vi "voltCtrl.vi"() -> ()   [LabVIEW 2023]
uses:
  <vilib>/DAQmx/write.llb/DAQmx Write (Analog 1D DBL NChan 1Samp).vi
  <vilib>/DAQmx/create/channels.llb/DAQmx Create Channel (AO-Voltage-Basic).vi
  <vilib>/DAQmx/miscellaneous.llb/DAQmx Fill In Error Info.vi
panel:
  out "?":bool
  in  "crr":bool
  in  "Input":dbl(slide) scale=0.0..5.0
  in  "vltg":bool
  out "?":bool
  in  "?":bool
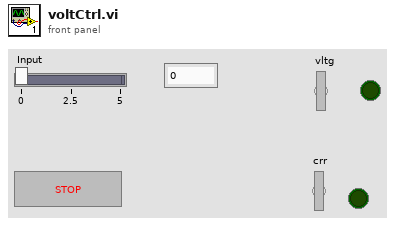
[diagram p1: front panel]
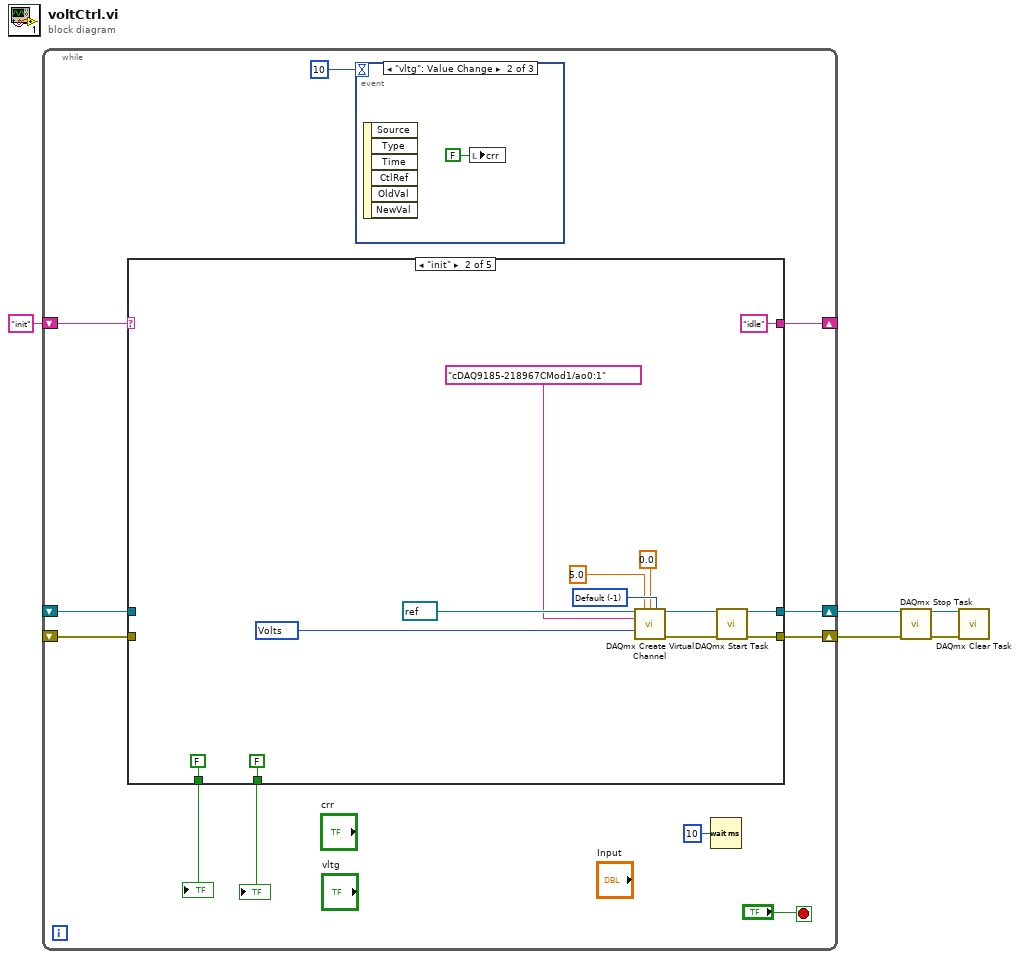
[diagram p0: block diagram]
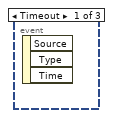
[diagram p2: hidden frame]
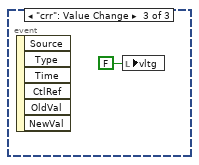
[diagram p3: hidden frame]
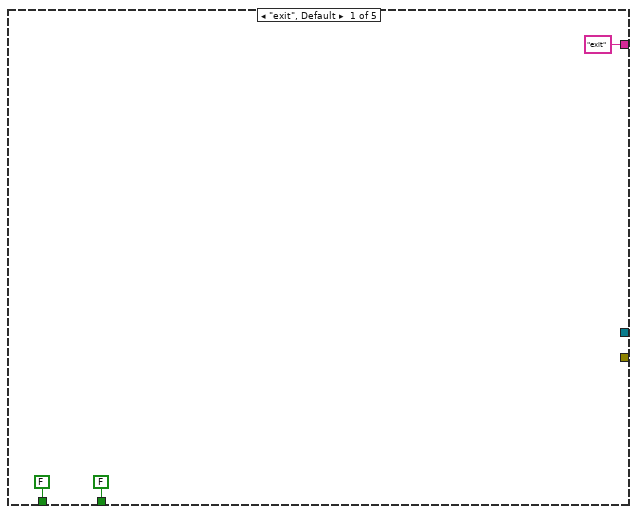
[diagram p4: hidden frame]
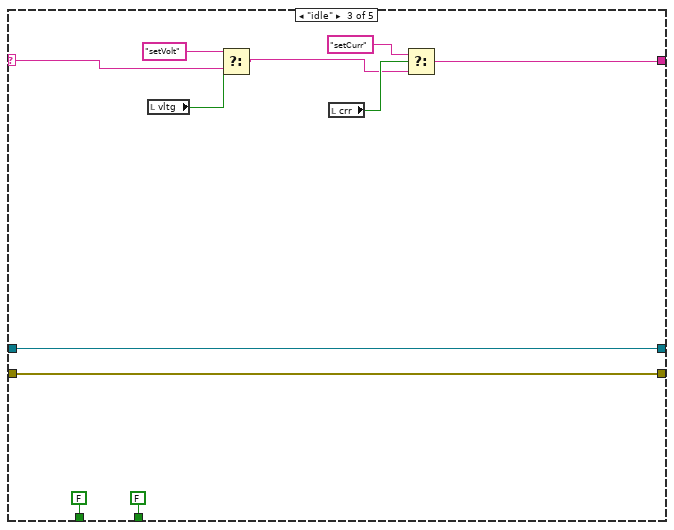
[diagram p5: hidden frame]
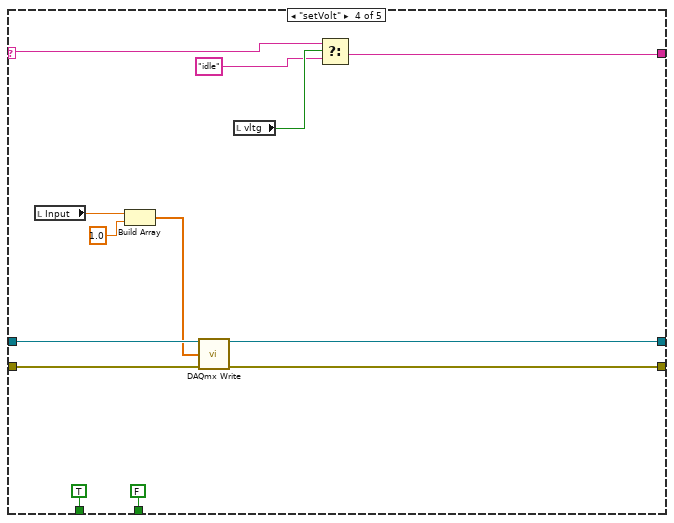
[diagram p6: hidden frame]
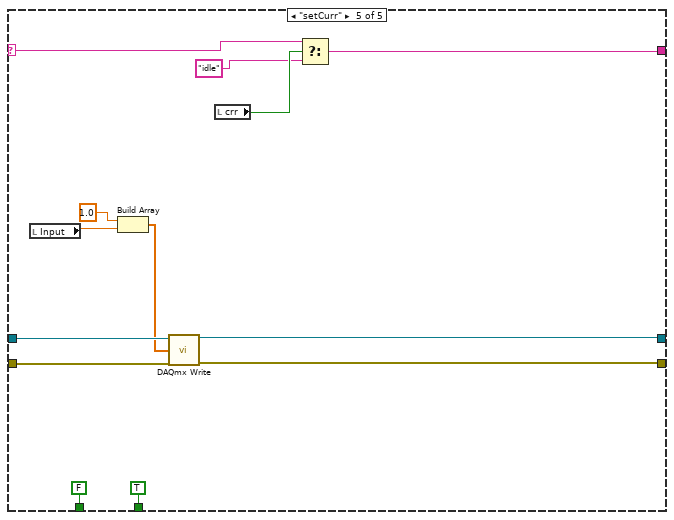
[diagram p7: hidden frame]
diagram:
  n1 = while {
    shift-right: [w15] -> _
    shift-left: "init" -> [w16]
    shift-right: [w14] -> w3
    shift-left: _ -> [w12]
    shift-right: [w13] -> w2
    shift-left: _ -> [w11]
    stop <- "?" stop-if-true
    n2 = case shown="\"init\"" w16 {
      selector: w16 -> [_ _ w41 w56 w63]
      tunnel: ["exit" "idle" w36 w54 w65] -> w15
      tunnel: [_ w31 w45 w51 w69] -> w14
      tunnel: [_ w30 w44 w50 w68] -> w13
      tunnel: w12 -> [_ _ w45 w53 w71]
      tunnel: w11 -> [_ _ w44 w52 w70]
      tunnel: [FALSE ("voltage") FALSE ("voltage") FALSE ("voltage") TRUE ("voltage") FALSE ("voltage")] -> w10
      tunnel: [FALSE ("voltage") FALSE ("voltage") FALSE ("voltage") FALSE ("voltage") TRUE ("voltage")] -> w6
      frame "exit", Default {
      }
      frame "init" {
        w32 = 10348 items=["Volts"=10348, "From Custom Scale"=10065] ("units")
        w33 = -1 items=["Default"=-1, "RSE"=10083, "Differential"=10106, "Pseudodifferential"=12529] ("output terminal configuration")
        n3 = call-poly <vilib>:"DAQmx Create Virtual Channel.vi"("task in"=refnum<k21> refnum, "maximum value"=5.0, "minimum value"=0.0, "output terminal configuration"=w33, "physical channels"=tag "cDAQ9185-218967CMod1/ao0:1", "units"=w32) -> ("task out"=w27:refnum<k21>, "error out"=w26:errorcluster)  [unwired: 8 in]
        n4 = call <vilib>:"DAQmx Start Task.vi"("task/channels in"=w27, "error in"=w26) -> ("task out"=w31:refnum<k21>, "error out"=w30:errorcluster)  [unwired: 12 in]
      }
      frame "idle" {
        n5 = local read "vltg"() -> (w40:bool)
        n6 = Select(t="setVolt", s=w40, f=w41) -> (s? t:f=w38:string)
        n7 = local read "crr"() -> (w39:bool)
        n8 = Select(t="setCurr", s=w39, f=w38) -> (s? t:f=w36:string)
      }
      frame "setVolt" {
        n9 = local read "Input"() -> (w47:dbl)
        n10 = Build Array(w47, 1.0 ("element")) -> (w48:dbl[])
        n11 = call-poly <vilib>:"DAQmx Write.vi"("task/channels in"=w53, "data"=w48, "error in"=w52) -> ("task out"=w51:refnum<k21>, "error out"=w50:errorcluster)  [unwired: 10 in, 1 out]
        n12 = local read "vltg"() -> (w57:bool)
        n13 = Select(t=w56, s=w57, f="idle") -> (s? t:f=w54:string)
      }
      frame "setCurr" {
        n14 = local read "Input"() -> (w61:dbl)
        n15 = Build Array(1.0 ("element"), w61) -> (w59:dbl[])
        n16 = call-poly <vilib>:"DAQmx Write.vi"("task/channels in"=w71, "data"=w59, "error in"=w70) -> ("task out"=w69:refnum<k21>, "error out"=w68:errorcluster)  [unwired: 10 in, 1 out]
        n17 = local read "crr"() -> (w64:bool)
        n18 = Select(t=w63, s=w64, f="idle") -> (s? t:f=w65:string)
      }
    }
    "?" <- w10
    "?" <- w6
    n19 = event shown="[1] \"vltg\": Value Change" {
      selector: _ -> [_ _ _]
      dyn-events: _ -> [_ _ _]
      timeout: 10 -> [_ _ _]
      event Timeout {
        n20 = event-data() -> ()  [unwired: 1 in, 3 out]
      }
      event "vltg": Value Change {
        n21 = event-data() -> ()  [unwired: 1 in, 6 out]
        n22 = local write "crr"(FALSE ("crr")) -> ()
      }
      event "crr": Value Change {
        n23 = event-data() -> ()  [unwired: 1 in, 6 out]
        n24 = local write "vltg"(FALSE ("vltg")) -> ()
      }
    }
    n25 = Wait (ms)(milliseconds to wait=u32 10 ("millisecond multiple")) -> ()  [unwired: 1 out]
  }
  n26 = call <vilib>:"DAQmx Stop Task.vi"("task/channels in"=w3, "error in"=w2) -> ("task out"=w5:refnum<k21>, "error out"=w4:errorcluster)  [unwired: 12 in]
  n27 = call <vilib>:"DAQmx Clear Task.vi"("task in"=w5, "error in"=w4) -> ()  [unwired: 13 in, 1 out]
